vi "setName.vi"(0 "reference":refnum<class "StateNode.lvclass">, 1 "name":refnum<class "MultiLineString.lvclass">, 5 "error in (no error)":errorcluster) -> (14 "reference out":refnum<class "StateNode.lvclass">, 19 "error out":errorcluster)   [LabVIEW 2012, in "StateNode.lvclass"]
doc: "public void setName(MultiLineString newValue)"
uses:
  <resource>/Framework/Providers/Open_GDS/UML/StateNode_class/StateNode.lvclass
  <resource>/Framework/Providers/Open_GDS/UML/MultiLineString_class/MultiLineString.lvclass
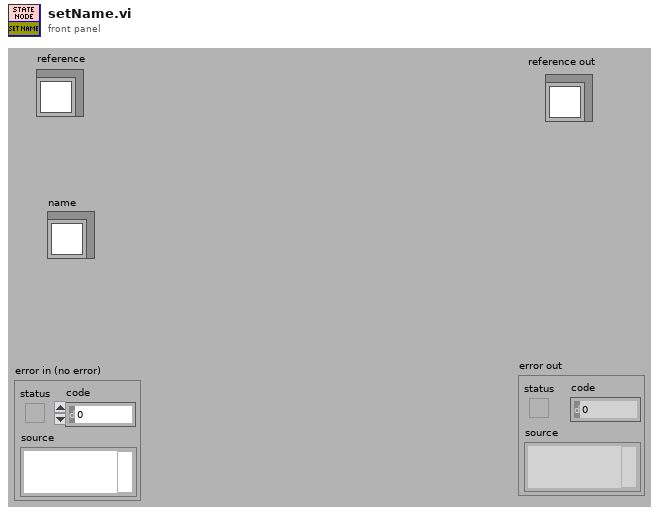
[diagram p1: front panel]
types:
  T1 = typedef "StateNode.lvclass/ObjectAttributes.ctl" = cluster{"Base class":T2, "state":refnum<class "MultiLineString.lvclass">, "action":refnum<class "MultiLineString.lvclass">, "DEFAULT_WIDTH":i32, "DEFAULT_HEIGHT":i32}
  T2 = typedef "RectangularNode.lvclass/ObjectAttributes.ctl" = cluster{"Base class":T3, "bounds":T4}
  T3 = typedef "AbstractNode.lvclass/ObjectAttributes.ctl" = cluster{"parent":refnum<class "AbstractNode.lvclass">, "children":refnum<class "AbstractNode.lvclass">[], "Hidden":bool}
  T4 = typedef "Rectangle Rectangle2D.ctl" = cluster{"x":dbl, "y":dbl, "width":dbl, "height":dbl}
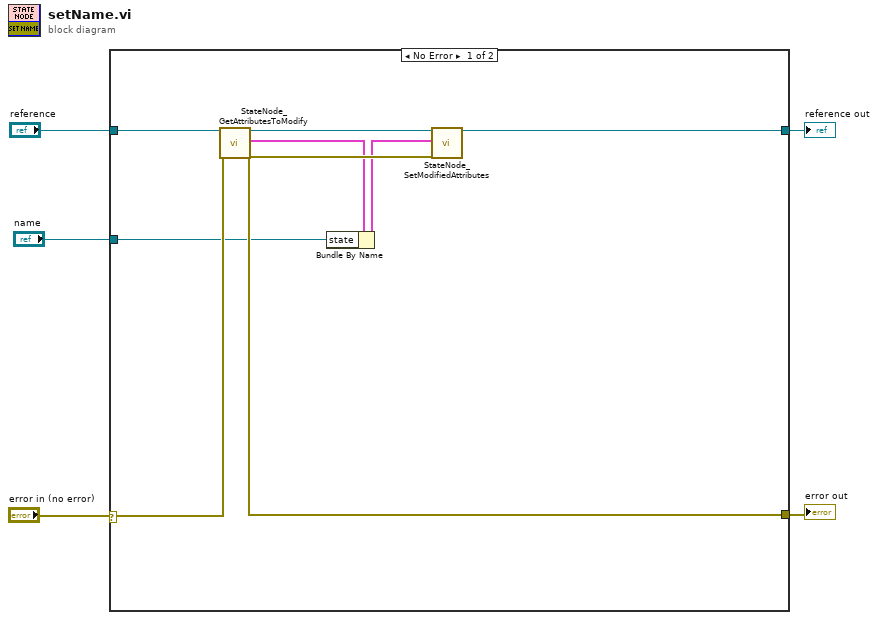
[diagram p0: block diagram]
diagram:
  n1 = case shown="No Error" "error in (no error)" {
    selector: "error in (no error)" -> [w9 w13]
    tunnel: "reference" -> [w12 w14]
    tunnel: [w11 w13] -> w4
    tunnel: [w10 w14] -> w3
    tunnel: "name" -> [w8 _]
    frame No Error {
      n2 = call <resource>:"StateNode_GetAttributesToModify.vi"("reference in"=w12, "error in (no error)"=w9) -> ("reference out"=w10:refnum<class "StateNode.lvclass">, "Attributes"=w6:T1, "error out"=w11:errorcluster)  [unwired: 1 in, 14 out]
      n3 = Bundle By Name(cluster=w6, "state"=w8) -> (w7:T1)
      n4 = call <resource>:"StateNode_SetModifiedAttributes.vi"("reference in"=w10, "Attributes"=w7, "error in (no error)"=w11) -> ()  [unwired: 3 in, 14 out]
    }
    frame Error {
    }
  }
  "reference out" <- w3
  "error out" <- w4
